vi "Connect to Web Stream.vi"() -> (0 "error out":errorcluster, 2 "Connected?":bool, 3 "Writer Endpoint":refnum<k21>)   [LabVIEW 2014]
uses:
  controls/UI DataSam.ctl
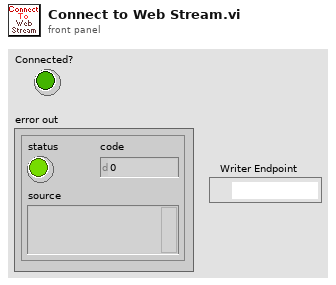
[diagram p1: front panel]
types:
  T1 = typedef "UI DataSam.ctl" = cluster{"Message":string, "Data":variant}
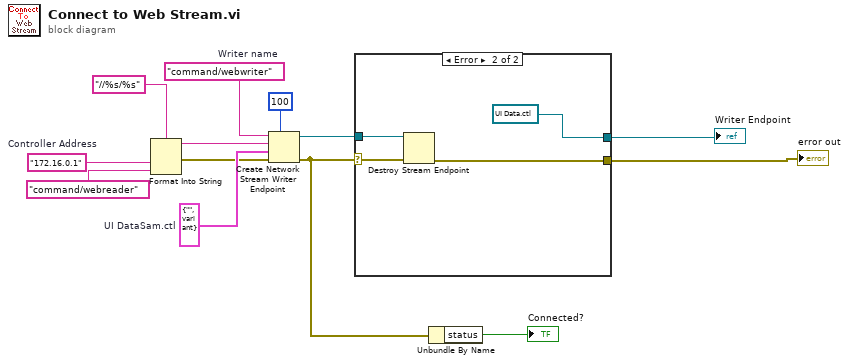
[diagram p0: block diagram]
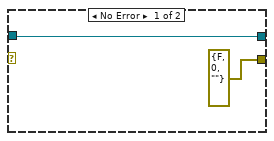
[diagram p2: hidden frame]
diagram:
  w11 = "172.16.0.1"  # Controller Address
  w7 = T1 {"Message"="", "Data"=variant}  # UI DataSam.ctl
  w6 = "command/webwriter"  # Writer name
  n1 = Format Into String(format string="//%s/%s", w11, "command/webreader" ("input 2")) -> (resulting string=w4:string, error out=w3:errorcluster)  [unwired: 2 in]
  n2 = Create Network Stream Writer Endpoint(7:100 ("writer buffer size"), 8:w3, 9:w7, 10:w4, 11:w6) -> (0:w9:errorcluster, 3:w8:refnum<k21>)  [unwired: 2 in]
  n3 = case shown="Error" w9 {
    selector: w9 -> [_ w19]
    tunnel: w8 -> [w15 w18]
    tunnel: [w15 refnum<k21> refnum ("Writer name")] -> w13
    tunnel: [errorcluster {"status"=FALSE, "code"=0, "source"=""} ("error out") w16] -> w10
    frame No Error {
    }
    frame Error {
      n4 = Destroy Stream Endpoint(8:w19, 11:w18) -> (0:w16:errorcluster)
    }
  }
  "error out" <- w10
  "Writer Endpoint" <- w13
  n5 = Unbundle By Name(w9) -> ("status"=→"Connected?":bool)
